vi "Check Color Table Size.vi"(1 "error in (no error)":errorcluster, 2 "depth":u8, 3 "color table":u32[](array[numeric])) -> (0 "error out":errorcluster)   [LabVIEW 2020]
doc: "Takes a bit depth and checks to be sure the color table is at least 2^depth elements in size."
uses:
  Error Cluster From Error Code.vi
  Error Ring.xnode
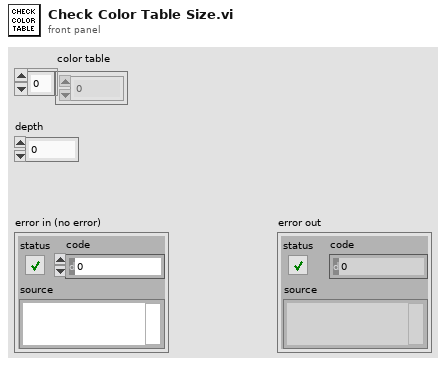
[diagram p1: front panel]
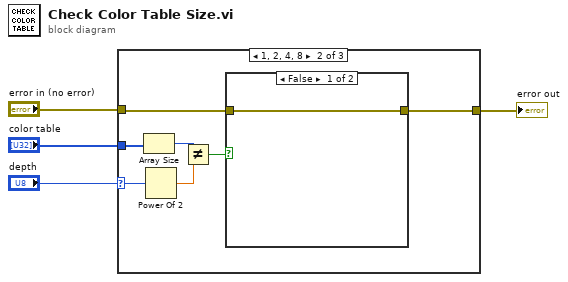
[diagram p0: block diagram]
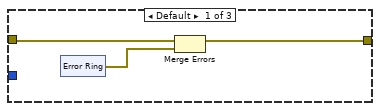
[diagram p2: hidden frame]
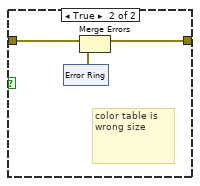
[diagram p3: hidden frame]
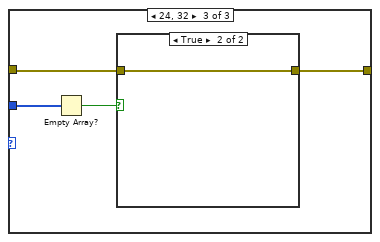
[diagram p4: hidden frame]
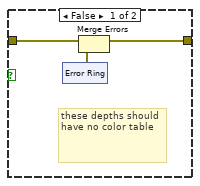
[diagram p5: hidden frame]
diagram:
  n1 = case shown="1, 2, 4, 8" "depth" {
    selector: "depth" -> [_ w12 _]
    tunnel: "color table" -> [_ w18 w28]
    tunnel: "error in (no error)" -> [w7 w14 w30]
    tunnel: [w6 w13 w29] -> w2
    frame Default {
      n2 = xnode "Error Ring"() -> ("error out"=w5:errorcluster)
      n3 = Merge Errors(w7, w5) -> (w6:errorcluster)
    }
    frame 1, 2, 4, 8 {
      n4 = Array Size(array=w18) -> (size(s)=w16:i32)
      n5 = Power Of 2(x=w12) -> (2^x=w17:dbl)
      n6 = Not Equal?(x=w16, y=w17) -> (x != y?=w15:bool)
      n7 = case shown="False" w15 {
        tunnel: w14 -> [w19 w22]
        tunnel: [w19 w21] -> w13
        frame False {
        }
        frame True {
          # "color table is wrong size"
          n8 = xnode "Error Ring"() -> ("error out"=w20:errorcluster)
          n9 = Merge Errors(w22, w20) -> (w21:errorcluster)
        }
      }
    }
    frame 24, 32 {
      n10 = Empty Array?(array=w28) -> (empty?=w27:bool)
      n11 = case shown="True" w27 {
        tunnel: w30 -> [w33 w38]
        tunnel: [w32 w38] -> w29
        frame False {
          # "these depths should have no color table"
          n12 = xnode "Error Ring"() -> ("error out"=w31:errorcluster)
          n13 = Merge Errors(w33, w31) -> (w32:errorcluster)
        }
        frame True {
        }
      }
    }
  }
  "error out" <- w2
